vi "XNET.Settings.vi"(6 "Action":enum8{"Get", "Set"}(ring), 8 "error in (no error)":errorcluster, 10 "XNET Settings":T1={"Database"="", "Cluster"="", "Primary"={"Port"="", "Baud Rate"=500000, "Termination"=1, "CAN I/O Mode"=0, "FD Baud Rate"=500000, "Priority"=100, "FD ISO Mode"=0}, "Ghost"={"Port"="", "Baud Rate"=0, "Termination"=0, "CAN I/O Mode"=0, "FD Baud Rate"=500000, "Priority"=100, "FD ISO Mode"=0}} {"Ghost"."FD ISO Mode" items=["ISO", "Non ISO", "ISO Legacy"]; "Ghost"."CAN I/O Mode" items=["CAN 2.0", "CAN FD", "CAN FD+BRS"]; "Ghost"."Termination" items=["Off", "On"]; "Primary"."FD ISO Mode" items=["ISO", "Non ISO", "ISO Legacy"]; "Primary"."CAN I/O Mode" items=["CAN 2.0", "CAN FD", "CAN FD+BRS"]; "Primary"."Termination" items=["Off", "On"]}, 11 "Parent Ref in":T3 format="%.0x") -> (0 "error out":errorcluster, 2 "XNET Settings":T1={"Database"="", "Cluster"="", "Primary"={"Port"="", "Baud Rate"=500000, "Termination"=1, "CAN I/O Mode"=0, "FD Baud Rate"=500000, "Priority"=100, "FD ISO Mode"=0}, "Ghost"={"Port"="", "Baud Rate"=0, "Termination"=0, "CAN I/O Mode"=0, "FD Baud Rate"=500000, "Priority"=100, "FD ISO Mode"=0}} {"Ghost"."FD ISO Mode" items=["ISO", "Non ISO", "ISO Legacy"]; "Ghost"."CAN I/O Mode" items=["CAN 2.0", "CAN FD", "CAN FD+BRS"]; "Ghost"."Termination" items=["Off", "On"]; "Primary"."FD ISO Mode" items=["ISO", "Non ISO", "ISO Legacy"]; "Primary"."CAN I/O Mode" items=["CAN 2.0", "CAN FD", "CAN FD+BRS"]; "Primary"."Termination" items=["Off", "On"]}, 3 "Item Ref out":T3 format="%.0x")   [LabVIEW 2019, in "Ghost Bus Addon System Explorer.lvlib"]
uses:
  Ghost Bus Addon System Explorer.lvlib
  <vilib>/NI VeriStand/Custom Device API/Custom Device API.lvlib
  <vilib>/NI VeriStand/Custom Device API/Get Item Property (String).vi
  <vilib>/NI VeriStand/Custom Device API/Get Item Property (U32).vi
  <vilib>/NI/NI VeriStand Advanced SysDef API/SysDef API/Advanced System Definition.lvlib
  <vilib>/NI/NI VeriStand Advanced SysDef API/_SubVIs/SysDef.Property.Set.String.vi
  <vilib>/NI/NI VeriStand Advanced SysDef API/_SubVIs/SysDef.Property.Set.U32.vi
  Addon Shared/SubVIs/GUID Lookup.vi
  Addon Shared/Ghost Bus Addon Shared.lvlib
  <vilib>/NI/NI VeriStand Advanced SysDef API/_SubVIs/SysDef.Property.Set.Variant.vi
  <vilib>/NI VeriStand/Custom Device API/Get Item Property (Variant).vi
  <vilib>/NI VeriStand/Custom Device API/Get Item Property (I32).vi
  <vilib>/NI/NI VeriStand Advanced SysDef API/_SubVIs/SysDef.Property.Set.I32.vi
  <vilib>/NI VeriStand/Custom Device API/Custom Device Item Ref.ctl
  Addon Shared/Types/XNET Settings.ctl
  Addon Shared/Types/XNET Port Settings.ctl
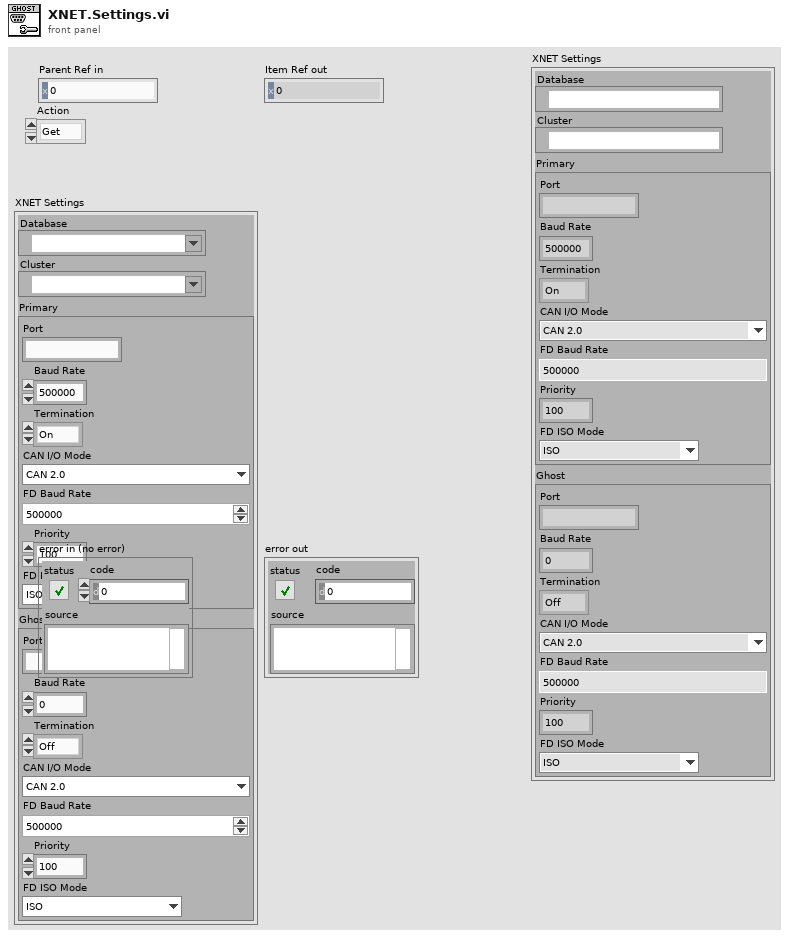
[diagram p1: front panel]
types:
  T1 = typedef "Ghost Bus Addon Shared.lvlib/XNET Settings.ctl" = cluster{"Database":refnum<k21>, "Cluster":refnum<k21>, "Primary":T2, "Ghost":T2}
  T2 = typedef "Ghost Bus Addon Shared.lvlib/XNET Port Settings.ctl" = cluster{"Port":string, "Baud Rate":u64, "Termination":u32, "CAN I/O Mode":u32, "FD Baud Rate":u64, "Priority":i32, "FD ISO Mode":u32}
  T3 = typedef "Custom Device API.lvlib/Custom Device Item Ref.ctl" = u64
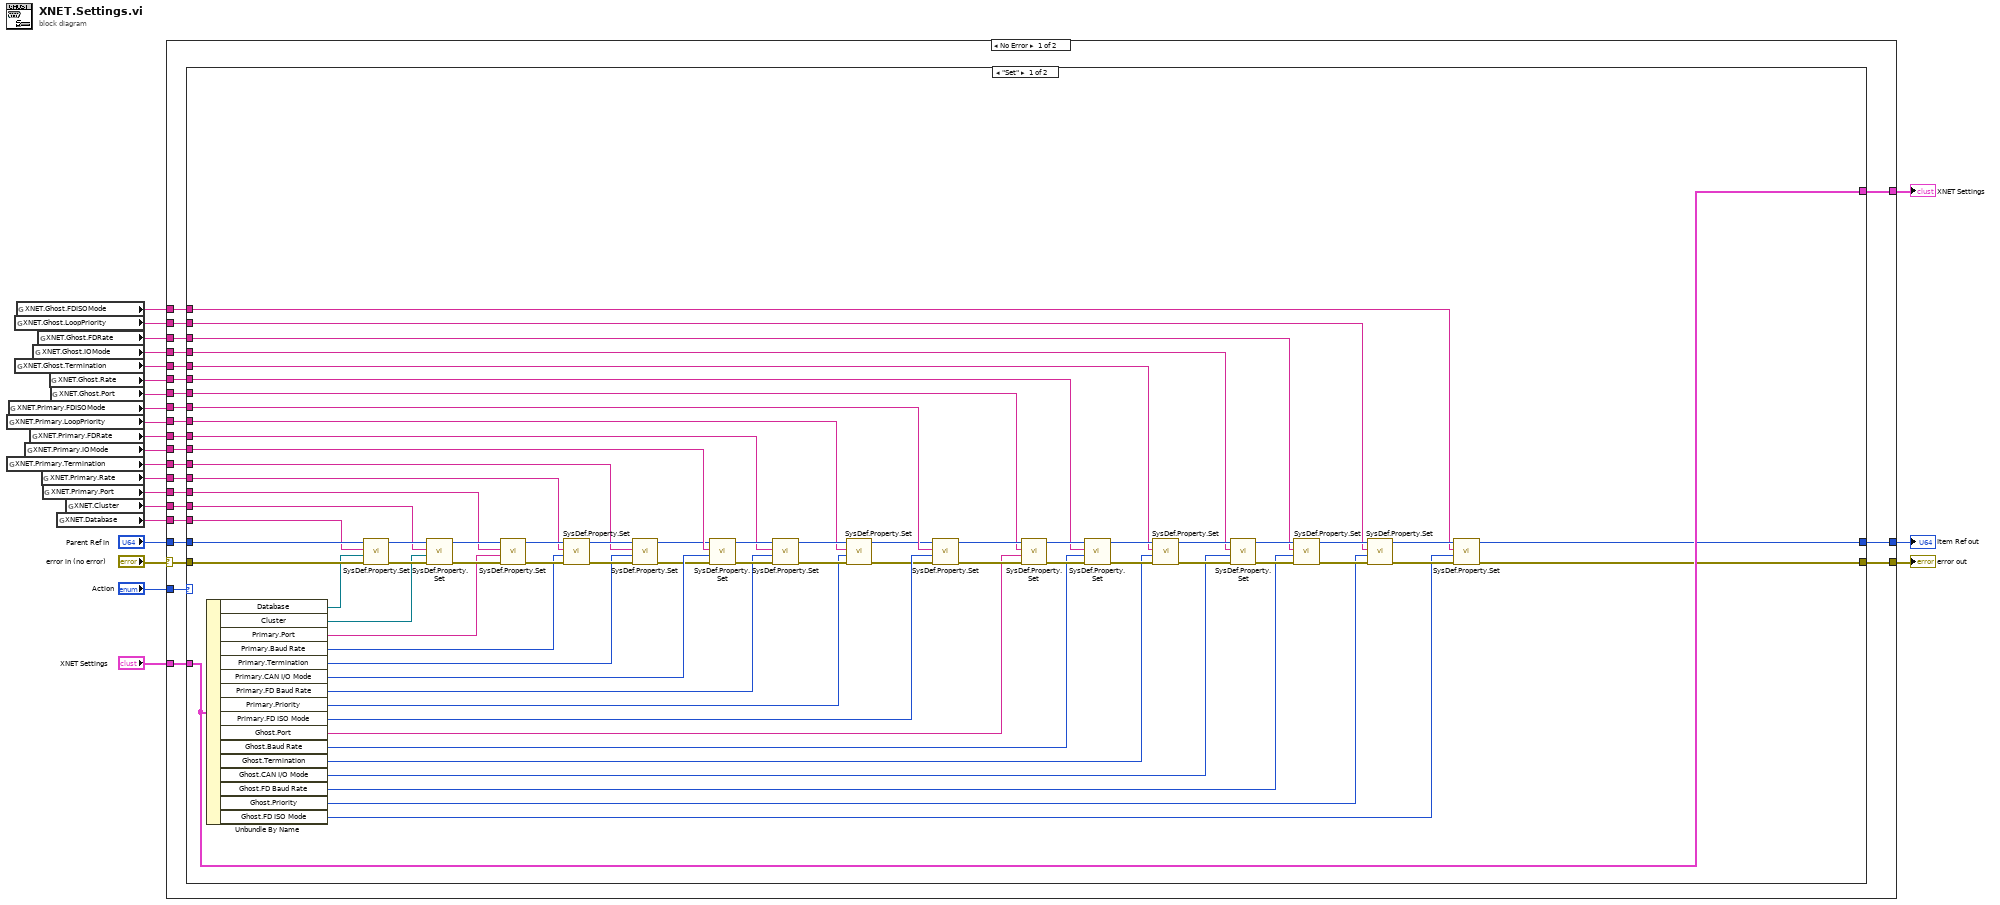
[diagram p0: block diagram]
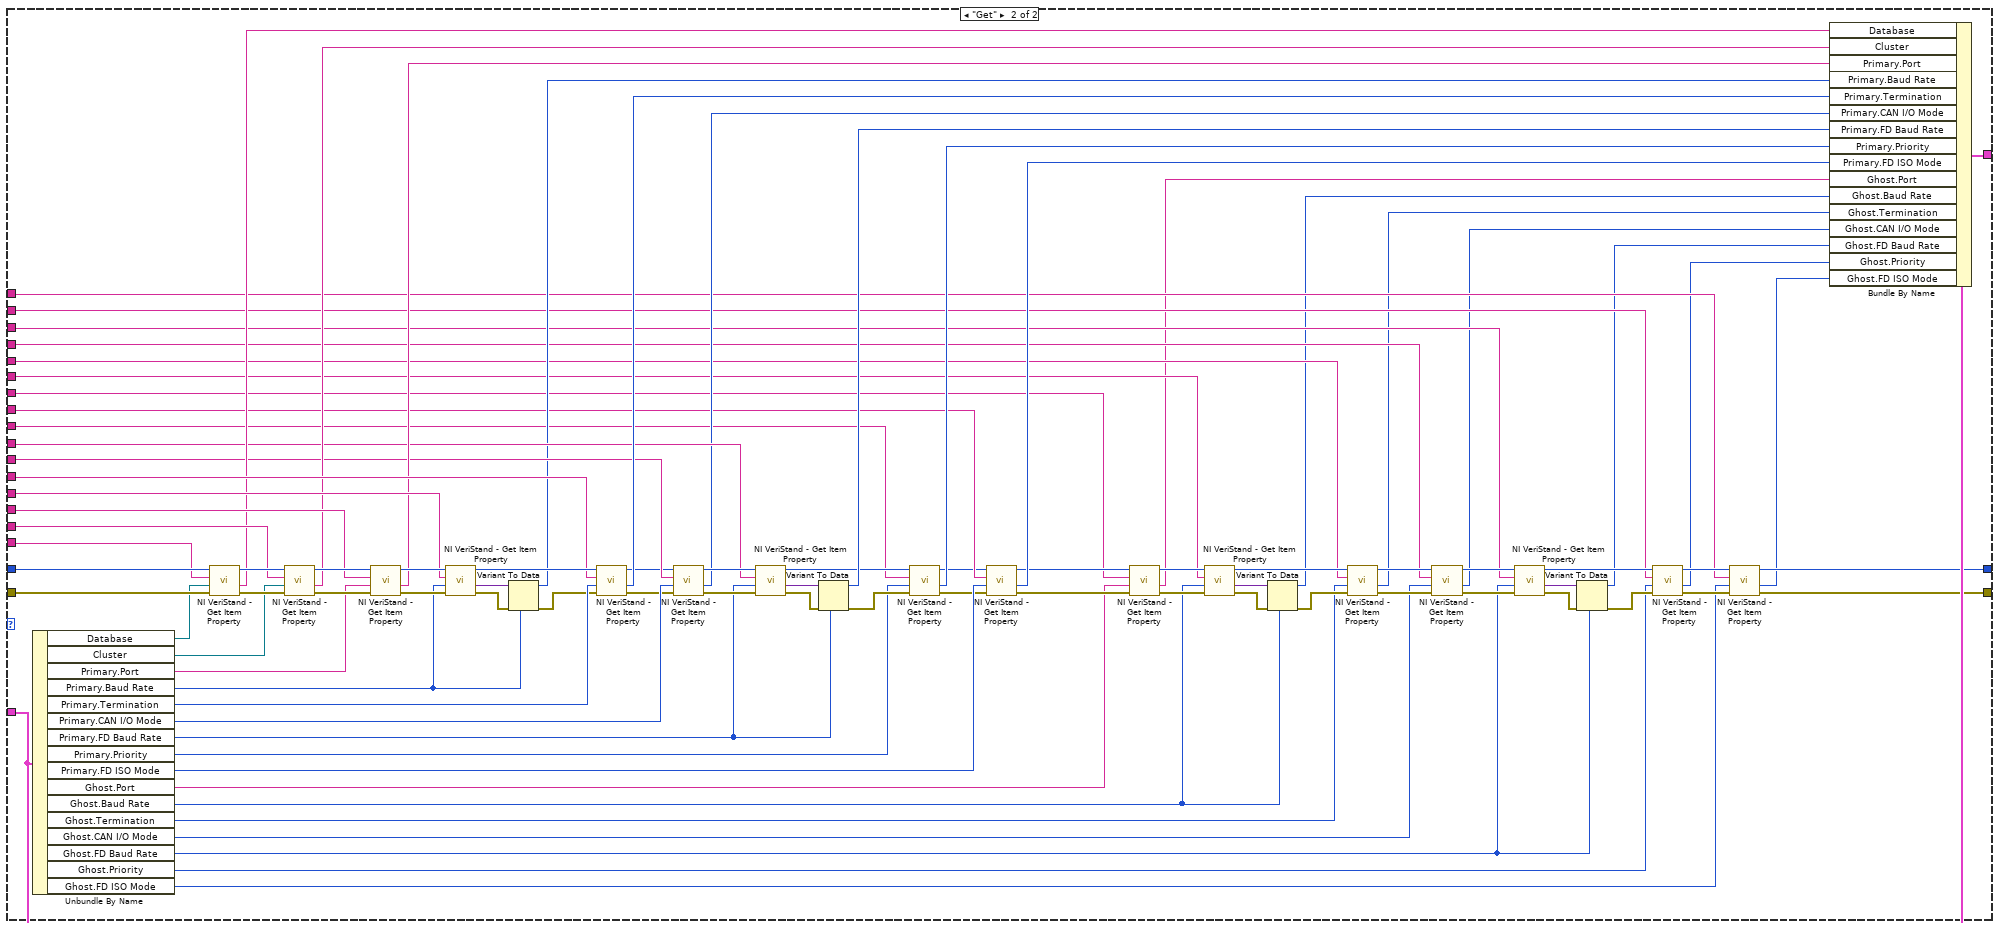
[diagram p2: hidden frame]
diagram:
  n1 = global read "GUID Lookup.vi" "XNET.Primary.LoopPriority"() -> (w9:string)
  n2 = global read "GUID Lookup.vi" "XNET.Primary.Termination"() -> (w12:string)
  n3 = global read "GUID Lookup.vi" "XNET.Primary.FDISOMode"() -> (w8:string)
  n4 = global read "GUID Lookup.vi" "XNET.Ghost.LoopPriority"() -> (w2:string)
  n5 = global read "GUID Lookup.vi" "XNET.Ghost.Termination"() -> (w5:string)
  n6 = global read "GUID Lookup.vi" "XNET.Ghost.FDISOMode"() -> (w1:string)
  n7 = global read "GUID Lookup.vi" "XNET.Primary.IOMode"() -> (w11:string)
  n8 = global read "GUID Lookup.vi" "XNET.Primary.FDRate"() -> (w10:string)
  n9 = global read "GUID Lookup.vi" "XNET.Ghost.IOMode"() -> (w4:string)
  n10 = global read "GUID Lookup.vi" "XNET.Ghost.FDRate"() -> (w3:string)
  n11 = global read "GUID Lookup.vi" "XNET.Primary.Rate"() -> (w13:string)
  n12 = global read "GUID Lookup.vi" "XNET.Primary.Port"() -> (w14:string)
  n13 = global read "GUID Lookup.vi" "XNET.Ghost.Rate"() -> (w6:string)
  n14 = global read "GUID Lookup.vi" "XNET.Ghost.Port"() -> (w7:string)
  n15 = global read "GUID Lookup.vi" "XNET.Database"() -> (w16:string)
  n16 = global read "GUID Lookup.vi" "XNET.Cluster"() -> (w15:string)
  n17 = case shown="No Error" "error in (no error)" {
    selector: "error in (no error)" -> [w37 w208]
    tunnel: "Parent Ref in" -> [w46 w207]
    tunnel: w16 -> [w45 _]
    tunnel: "XNET Settings" -> [w44 w206]
    tunnel: [w43 w208] -> w21
    tunnel: [w42 w207] -> w20
    tunnel: w15 -> [w41 _]
    tunnel: w14 -> [w40 _]
    tunnel: w12 -> [w39 _]
    tunnel: w13 -> [w38 _]
    tunnel: "Action" -> [w36 _]
    tunnel: [w35 w206] -> w17
    tunnel: w11 -> [w34 _]
    tunnel: w10 -> [w33 _]
    tunnel: w9 -> [w32 _]
    tunnel: w8 -> [w31 _]
    tunnel: w7 -> [w30 _]
    tunnel: w6 -> [w29 _]
    tunnel: w5 -> [w28 _]
    tunnel: w4 -> [w27 _]
    tunnel: w3 -> [w26 _]
    tunnel: w2 -> [w25 _]
    tunnel: w1 -> [w24 _]
    frame No Error {
      n18 = case shown="\"Set\"" w36 {
        tunnel: w46 -> [w113 w205]
        tunnel: w45 -> [w112 w204]
        tunnel: w44 -> [w94 w187]
        tunnel: [w62 w136] -> w43
        tunnel: [w61 w135] -> w42
        tunnel: w41 -> [w99 w196]
        tunnel: w40 -> [w98 w195]
        tunnel: w39 -> [w97 w194]
        tunnel: w38 -> [w96 w193]
        tunnel: w37 -> [w95 w192]
        tunnel: [w94 w182] -> w35
        tunnel: w34 -> [w90 w178]
        tunnel: w33 -> [w89 w177]
        tunnel: w32 -> [w81 w162]
        tunnel: w31 -> [w80 w159]
        tunnel: w30 -> [w53 w129]
        tunnel: w29 -> [w52 w128]
        tunnel: w28 -> [w51 w127]
        tunnel: w27 -> [w50 w126]
        tunnel: w26 -> [w49 w125]
        tunnel: w25 -> [w48 w124]
        tunnel: w24 -> [w47 w123]
        frame "Set" {
          n19 = Unbundle By Name(w94) -> ("Database"=w93:refnum<k21>, "Cluster"=w103:refnum<k21>, "Primary.Port"=w102:string, "Primary.Baud Rate"=w101:u64, "Primary.Termination"=w100:u32, "Primary.CAN I/O Mode"=w88:u32, "Primary.FD Baud Rate"=w87:u64, "Primary.Priority"=w82:i32, "Primary.FD ISO Mode"=w79:u32, "Ghost.Port"=w60:string, "Ghost.Baud Rate"=w59:u64, "Ghost.Termination"=w58:u32, "Ghost.CAN I/O Mode"=w57:u32, "Ghost.FD Baud Rate"=w56:u64, "Ghost.Priority"=w55:i32, "Ghost.FD ISO Mode"=w54:u32)
          n20 = call-poly <vilib>:"SysDef.Property.Set.vi"("error in (no error)"=w95, "Value"=w93, "Property Name"=w112, "nodeID"=w113) -> ("error out"=w109:errorcluster, "nodeID out"=w108:u64)  [unwired: 6 in]
          n21 = call-poly <vilib>:"SysDef.Property.Set.vi"("error in (no error)"=w109, "Value"=w103, "Property Name"=w99, "nodeID"=w108) -> ("error out"=w110:errorcluster, "nodeID out"=w111:u64)  [unwired: 6 in]
          n22 = call-poly <vilib>:"SysDef.Property.Set.vi"("error in (no error)"=w110, "Value"=w102, "Property Name"=w98, "nodeID"=w111) -> ("error out"=w105:errorcluster, "nodeID out"=w104:u64)  [unwired: 6 in]
          n23 = call-poly <vilib>:"SysDef.Property.Set.vi"("error in (no error)"=w105, "Value"=w101, "Property Name"=w96, "nodeID"=w104) -> ("error out"=w106:errorcluster, "nodeID out"=w107:u64)  [unwired: 6 in]
          n24 = call-poly <vilib>:"SysDef.Property.Set.vi"("error in (no error)"=w106, "Value"=w100, "Property Name"=w97, "nodeID"=w107) -> ("error out"=w86:errorcluster, "nodeID out"=w85:u64)  [unwired: 6 in]
          n25 = call-poly <vilib>:"SysDef.Property.Set.vi"("error in (no error)"=w86, "Value"=w88, "Property Name"=w90, "nodeID"=w85) -> ("error out"=w92:errorcluster, "nodeID out"=w91:u64)  [unwired: 6 in]
          n26 = call-poly <vilib>:"SysDef.Property.Set.vi"("error in (no error)"=w92, "Value"=w87, "Property Name"=w89, "nodeID"=w91) -> ("error out"=w84:errorcluster, "nodeID out"=w83:u64)  [unwired: 6 in]
          n27 = call-poly <vilib>:"SysDef.Property.Set.vi"("error in (no error)"=w84, "Value"=w82, "Property Name"=w81, "nodeID"=w83) -> ("error out"=w78:errorcluster, "nodeID out"=w77:u64)  [unwired: 6 in]
          n28 = call-poly <vilib>:"SysDef.Property.Set.vi"("error in (no error)"=w78, "Value"=w79, "Property Name"=w80, "nodeID"=w77) -> ("error out"=w64:errorcluster, "nodeID out"=w63:u64)  [unwired: 6 in]
          n29 = call-poly <vilib>:"SysDef.Property.Set.vi"("error in (no error)"=w64, "Value"=w60, "Property Name"=w53, "nodeID"=w63) -> ("error out"=w67:errorcluster, "nodeID out"=w68:u64)  [unwired: 6 in]
          n30 = call-poly <vilib>:"SysDef.Property.Set.vi"("error in (no error)"=w67, "Value"=w59, "Property Name"=w52, "nodeID"=w68) -> ("error out"=w66:errorcluster, "nodeID out"=w65:u64)  [unwired: 6 in]
          n31 = call-poly <vilib>:"SysDef.Property.Set.vi"("error in (no error)"=w66, "Value"=w58, "Property Name"=w51, "nodeID"=w65) -> ("error out"=w71:errorcluster, "nodeID out"=w72:u64)  [unwired: 6 in]
          n32 = call-poly <vilib>:"SysDef.Property.Set.vi"("error in (no error)"=w71, "Value"=w57, "Property Name"=w50, "nodeID"=w72) -> ("error out"=w69:errorcluster, "nodeID out"=w70:u64)  [unwired: 6 in]
          n33 = call-poly <vilib>:"SysDef.Property.Set.vi"("error in (no error)"=w69, "Value"=w56, "Property Name"=w49, "nodeID"=w70) -> ("error out"=w73:errorcluster, "nodeID out"=w74:u64)  [unwired: 6 in]
          n34 = call-poly <vilib>:"SysDef.Property.Set.vi"("error in (no error)"=w73, "Value"=w55, "Property Name"=w48, "nodeID"=w74) -> ("error out"=w75:errorcluster, "nodeID out"=w76:u64)  [unwired: 6 in]
          n35 = call-poly <vilib>:"SysDef.Property.Set.vi"("error in (no error)"=w75, "Value"=w54, "Property Name"=w47, "nodeID"=w76) -> ("error out"=w62:errorcluster, "nodeID out"=w61:u64)  [unwired: 6 in]
        }
        frame "Get" {
          n36 = Unbundle By Name(w187) -> ("Database"=w191:refnum<k21>, "Cluster"=w190:refnum<k21>, "Primary.Port"=w189:string, "Primary.Baud Rate"=w168:u64, "Primary.Termination"=w188:u32, "Primary.CAN I/O Mode"=w179:u32, "Primary.FD Baud Rate"=w174:u64, "Primary.Priority"=w161:i32, "Primary.FD ISO Mode"=w158:u32, "Ghost.Port"=w134:string, "Ghost.Baud Rate"=w115:u64, "Ghost.Termination"=w133:u32, "Ghost.CAN I/O Mode"=w132:u32, "Ghost.FD Baud Rate"=w114:u64, "Ghost.Priority"=w130:i32, "Ghost.FD ISO Mode"=w131:u32)
          n37 = call-poly <vilib>:"NI VeriStand - Get Item Property.vi"("error in (no error)"=w192, "Default Value"=w191, "Property Name"=w204, "Item Ref in"=w205) -> ("error out"=w201:errorcluster, "Value"=w186:string, "Item Ref out"=w200:T3)  [unwired: 4 in, 1 out]
          n38 = call-poly <vilib>:"NI VeriStand - Get Item Property.vi"("error in (no error)"=w201, "Default Value"=w190, "Property Name"=w196, "Item Ref in"=w200) -> ("error out"=w202:errorcluster, "Value"=w185:string, "Item Ref out"=w203:T3)  [unwired: 4 in, 1 out]
          n39 = call-poly <vilib>:"NI VeriStand - Get Item Property.vi"("error in (no error)"=w202, "Default Value"=w189, "Property Name"=w195, "Item Ref in"=w203) -> ("error out"=w198:errorcluster, "Value"=w184:string, "Item Ref out"=w197:T3)  [unwired: 4 in, 1 out]
          n40 = call-poly <vilib>:"NI VeriStand - Get Item Property.vi"("error in (no error)"=w198, "Default Value"=w168, "Property Name"=w193, "Item Ref in"=w197) -> ("error out"=w165:errorcluster, "Value"=w167:variant, "Item Ref out"=w199:T3)  [unwired: 4 in, 1 out]
          n41 = Variant To Data(error in=w165, type=w168, Variant=w167) -> (data=w166:u64, error out=w169:errorcluster)
          n42 = call-poly <vilib>:"NI VeriStand - Get Item Property.vi"("error in (no error)"=w169, "Default Value"=w188, "Property Name"=w194, "Item Ref in"=w199) -> ("error out"=w170:errorcluster, "Value"=w183:u32, "Item Ref out"=w171:T3)  [unwired: 4 in, 1 out]
          n43 = call-poly <vilib>:"NI VeriStand - Get Item Property.vi"("error in (no error)"=w170, "Default Value"=w179, "Property Name"=w178, "Item Ref in"=w171) -> ("error out"=w181:errorcluster, "Value"=w176:u32, "Item Ref out"=w180:T3)  [unwired: 4 in, 1 out]
          n44 = call-poly <vilib>:"NI VeriStand - Get Item Property.vi"("error in (no error)"=w181, "Default Value"=w174, "Property Name"=w177, "Item Ref in"=w180) -> ("error out"=w173:errorcluster, "Value"=w175:variant, "Item Ref out"=w163:T3)  [unwired: 4 in, 1 out]
          n45 = Variant To Data(error in=w173, type=w174, Variant=w175) -> (data=w172:u64, error out=w164:errorcluster)
          n46 = call-poly <vilib>:"NI VeriStand - Get Item Property.vi"("error in (no error)"=w164, "Default Value"=w161, "Property Name"=w162, "Item Ref in"=w163) -> ("error out"=w156:errorcluster, "Value"=w160:i32, "Item Ref out"=w155:T3)  [unwired: 4 in, 1 out]
          n47 = call-poly <vilib>:"NI VeriStand - Get Item Property.vi"("error in (no error)"=w156, "Default Value"=w158, "Property Name"=w159, "Item Ref in"=w155) -> ("error out"=w138:errorcluster, "Value"=w157:u32, "Item Ref out"=w137:T3)  [unwired: 4 in, 1 out]
          n48 = call-poly <vilib>:"NI VeriStand - Get Item Property.vi"("error in (no error)"=w138, "Default Value"=w134, "Property Name"=w129, "Item Ref in"=w137) -> ("error out"=w140:errorcluster, "Value"=w122:string, "Item Ref out"=w141:T3)  [unwired: 4 in, 1 out]
          n49 = call-poly <vilib>:"NI VeriStand - Get Item Property.vi"("error in (no error)"=w140, "Default Value"=w115, "Property Name"=w128, "Item Ref in"=w141) -> ("error out"=w150:errorcluster, "Value"=w149:variant, "Item Ref out"=w139:T3)  [unwired: 4 in, 1 out]
          n50 = Variant To Data(error in=w150, type=w115, Variant=w149) -> (data=w121:u64, error out=w148:errorcluster)
          n51 = call-poly <vilib>:"NI VeriStand - Get Item Property.vi"("error in (no error)"=w148, "Default Value"=w133, "Property Name"=w127, "Item Ref in"=w139) -> ("error out"=w147:errorcluster, "Value"=w120:u32, "Item Ref out"=w146:T3)  [unwired: 4 in, 1 out]
          n52 = call-poly <vilib>:"NI VeriStand - Get Item Property.vi"("error in (no error)"=w147, "Default Value"=w132, "Property Name"=w126, "Item Ref in"=w146) -> ("error out"=w142:errorcluster, "Value"=w119:u32, "Item Ref out"=w143:T3)  [unwired: 4 in, 1 out]
          n53 = call-poly <vilib>:"NI VeriStand - Get Item Property.vi"("error in (no error)"=w142, "Default Value"=w114, "Property Name"=w125, "Item Ref in"=w143) -> ("error out"=w145:errorcluster, "Value"=w144:variant, "Item Ref out"=w152:T3)  [unwired: 4 in, 1 out]
          n54 = Variant To Data(error in=w145, type=w114, Variant=w144) -> (data=w118:u64, error out=w151:errorcluster)
          n55 = call-poly <vilib>:"NI VeriStand - Get Item Property.vi"("error in (no error)"=w151, "Default Value"=w130, "Property Name"=w124, "Item Ref in"=w152) -> ("error out"=w153:errorcluster, "Value"=w117:i32, "Item Ref out"=w154:T3)  [unwired: 4 in, 1 out]
          n56 = call-poly <vilib>:"NI VeriStand - Get Item Property.vi"("error in (no error)"=w153, "Default Value"=w131, "Property Name"=w123, "Item Ref in"=w154) -> ("error out"=w136:errorcluster, "Value"=w116:u32, "Item Ref out"=w135:T3)  [unwired: 4 in, 1 out]
          n57 = Bundle By Name(cluster=w187, "Database"=w186, "Cluster"=w185, "Primary.Port"=w184, "Primary.Baud Rate"=w166, "Primary.Termination"=w183, "Primary.CAN I/O Mode"=w176, "Primary.FD Baud Rate"=w172, "Primary.Priority"=w160, "Primary.FD ISO Mode"=w157, "Ghost.Port"=w122, "Ghost.Baud Rate"=w121, "Ghost.Termination"=w120, "Ghost.CAN I/O Mode"=w119, "Ghost.FD Baud Rate"=w118, "Ghost.Priority"=w117, "Ghost.FD ISO Mode"=w116) -> (w182:T1)
        }
      }
    }
    frame Error {
    }
  }
  "Item Ref out" <- w20
  "error out" <- w21
  "XNET Settings" <- w17
